vi "LabJackU3_TC_Main.vi"() -> ()   [LabVIEW 2019]
uses:
  temperature_status_LabJackU3.ctl
  LabJackU3_Global.vi
panel:
  in  "LO":dbl
  in  "LOLO":dbl
  in  "HI":dbl=110.0
  in  "HIHI":dbl=115.0
  out "Temp. Status":T1
  out "status_log":bool caption="Status"
  in  "Logging":bool=TRUE
  in  "Device S/N":string="320107447"
  out "Loops Avg (V)":dbl format="%.6f"
  out "External CJC (F)":dbl format="%.1f"
  out "Internal CJC (F)":dbl format="%.1f"
  out "Message":string
  out "Temperature (F)":dbl[](array[numeric]) format="%.1f"
  out "Voltage (V)":dbl[](array[numeric])
  out "Readout Status":bool
  out "Chart B":waveform(dbl)[](graph)
  out "Chart A":waveform(dbl)[](graph)
  out "Last Meas. Time":timestamp format="%<%Y-%m-%d %H:%M:%S>T"
  in  "Meas. Interval":u32=30 caption="s"
  in  "Samples per Meas.":i32=500
  in  "stop":bool
  in  "Channel ID":i32[](array[numeric])=[2, 3, 4, 5, 6, 10, 11, 12, 13, 14, 30, 0, 7, 8, 9]
  # "QT Compressor Temperature"
  # "TC 1A"
  # "TC 2A"
  # "TC 3A"
  # "TC 4A"
  # "TC 5A"
  # "TC 1B"
  # "TC 2B"
  # "TC 3B"
  # "TC 4B"
  # "TC 5B"
  # "Internal CJC"
  # "External CJC"
  # "Loop 1"
  # "Loop 2"
  # "Loop 3"
  # "LabJack U3"
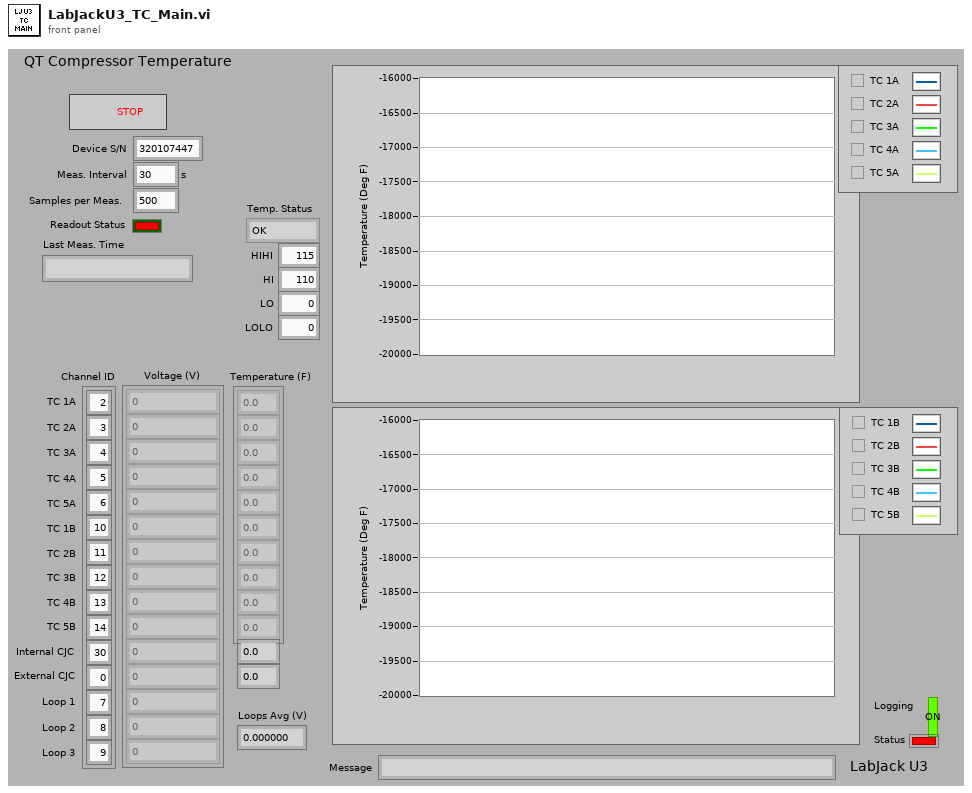
[diagram p1: front panel]
types:
  T1 = typedef "temperature_status_LabJackU3.ctl" = enum16{"OK", "UNKNOWN", "WARNING", "ERROR"}
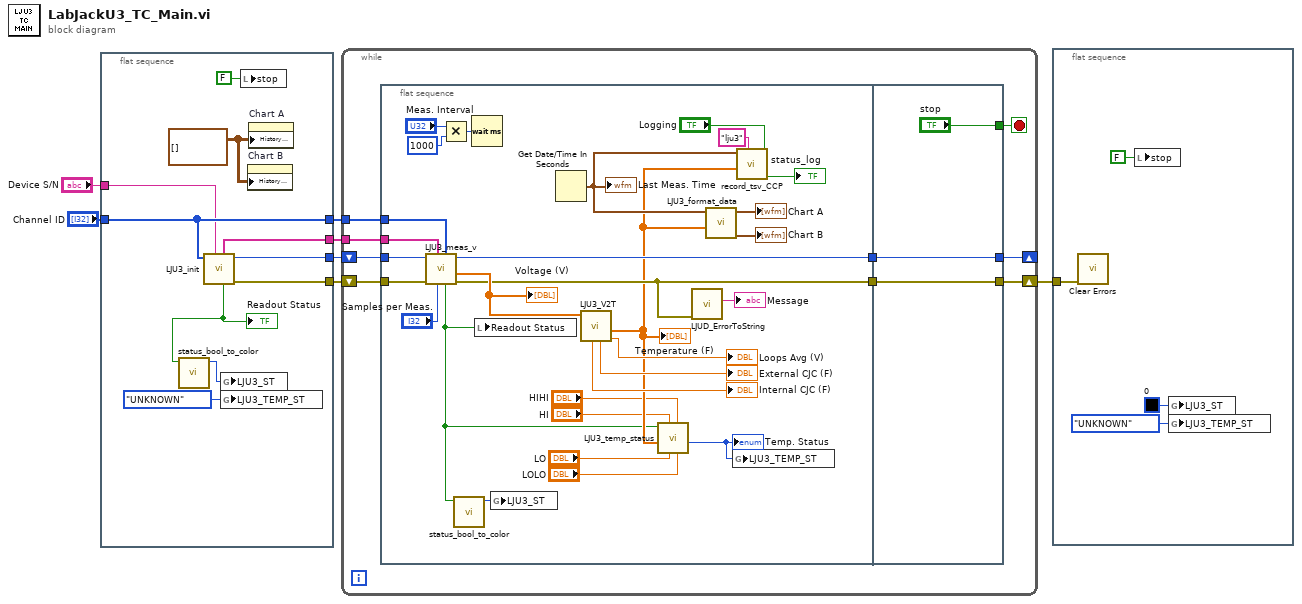
[diagram p0: block diagram]
diagram:
  n1 = flat-sequence {
    tunnel: [w17] -> w7
    tunnel: [w16] -> w6
    tunnel: [w15] -> w5
    tunnel: "Channel ID" -> [w13]
    tunnel: [w13] -> w3
    tunnel: "Device S/N" -> [w12]
    frame #0 {
      w14 = waveform(dbl)[][] [] ("History Data")
      n2 = call "LJU3_init.vi"("Address"=w12, "channel_list"=w13) -> ("error out"=w17:errorcluster, "handle"=w16:i32, "status"=w8:bool, "mode_list"=w15:string[])  [unwired: 6 in]
      "Readout Status" <- w8
      n3 = call "status_bool_to_color.vi"("status_bool_1"=w8) -> ("status_color"=w9:u32)  [unwired: 10 in]
      n4 = global write "LabJackU3_Global.vi" "LJU3_ST"(w9) -> ()
      n5 = global write "LabJackU3_Global.vi" "LJU3_TEMP_ST"(temperature_status_LabJackU3."UNKNOWN" ("LJU3_TEMP_ST")) -> ()
      n6 = local write "stop"(FALSE ("stop")) -> ()
      n7 = property on="Chart B" class="WFChart (strict)"("History Data"=w14) -> ()  [unwired: 2 in, 2 out]
      n8 = property on="Chart A" class="WFChart (strict)"("History Data"=w14) -> ()  [unwired: 2 in, 2 out]
    }
  }
  n9 = while {
    tunnel: w3 -> [w22]
    tunnel: w5 -> [w21]
    shift-right: [w23] -> w1
    shift-left: w7 -> [w26]
    shift-right: [w24] -> _
    shift-left: w6 -> [w25]
    stop <- w18 stop-if-true
    n10 = flat-sequence {
      tunnel: w26 -> [w55]
      tunnel: w25 -> [w54]
      tunnel: w22 -> [w48]
      tunnel: w21 -> [w47]
      tunnel: [w51] -> w20
      tunnel: [w50] -> w19
      tunnel: [w57] -> w23
      tunnel: [w58] -> w24
      tunnel: w20 -> [w58]
      tunnel: w19 -> [w57]
      tunnel: ["stop"] -> w18
      frame #0 {
        n11 = call "LJU3_meas_v.vi"("channel_list"=w48, "n_avg"="Samples per Meas.", "IOTypes"=w47, "error in"=w55, "handle in"=w54) -> ("error out"=w50:errorcluster, "array_voltage"=w53:dbl[], "handle out"=w51:i32, "status"=w31:bool)  [unwired: 3 in]
        "Voltage (V)" <- w53
        n12 = Multiply(x="Meas. Interval", y=u32 1000) -> (x*y=w29:u32)
        n13 = call "status_bool_to_color.vi"("status_bool_1"=w31) -> ("status_color"=w32:u32)  [unwired: 10 in]
        n14 = Wait (ms)(milliseconds to wait=w29) -> ()  [unwired: 1 out]
        n15 = local write "Readout Status"(w31) -> ()
        n16 = global write "LabJackU3_Global.vi" "LJU3_ST"(w32) -> ()
        n17 = Get Date/Time In Seconds() -> (seconds since 1Jan1904=w41:timestamp)
        "Last Meas. Time" <- w41
        n18 = call "LJU3_V2T.vi"("voltage_array"=w53) -> ("V_loop_mean"=→"Loops Avg (V)":dbl, "array_T_F"=w37:dbl[], "External CJC (F)"=→"External CJC (F)":dbl, "Internal CJC (F)"=→"Internal CJC (F)":dbl)  [unwired: 7 in]
        "Temperature (F)" <- w37
        n19 = call "LJU3_temp_status.vi"("lolo"="LOLO", "hihi"="HIHI", "lo"="LO", "hi"="HI", "T"=w37, "readout_status"=w31) -> ("temp_status"=w30:T1)  [unwired: 5 in]
        "Temp. Status" <- w30
        n20 = call "LJUD_ErrorToString.vi"("error in"=w50) -> ("String"=→"Message":string)  [unwired: 10 in]
        n21 = call "LJU3_format_data.vi"("value_array"=w37, "time"=w41) -> ("waveform_array_B"=→"Chart B":waveform(dbl)[], "waveform_array_A"=→"Chart A":waveform(dbl)[])  [unwired: 8 in]
        n22 = global write "LabJackU3_Global.vi" "LJU3_TEMP_ST"(w30) -> ()
        n23 = call "record_tsv_CCP.vi"("logging_on"="Logging", "folder_name"="lju3", "value_array"=w37, "time"=w41) -> ("status"=→"status_log":bool)  [unwired: 6 in, 1 out]
      }
      frame #1 {
      }
    }
  }
  n24 = flat-sequence {
    tunnel: w1 -> [w62]
    frame #0 {
      n25 = call <vilib>:"Clear Errors.vi"("error in (no error)"=w62) -> ()  [unwired: 5 in, 2 out]
      n26 = local write "stop"(FALSE ("stop")) -> ()
      n27 = global write "LabJackU3_Global.vi" "LJU3_ST"(u32 0 ("LJU3_ST")) -> ()
      n28 = global write "LabJackU3_Global.vi" "LJU3_TEMP_ST"(temperature_status_LabJackU3."UNKNOWN" ("LJU3_TEMP_ST")) -> ()
    }
  }
